vi "TwTpsGetModuleCodes.vi"(0 "error in (no error)":errorcluster) -> (1 "error out":errorcluster, 2 "moduleCodeBuffer":i32[](array[numeric]))   [LabVIEW 2009]
uses:
  Release_Build/TofDaqDll.dll
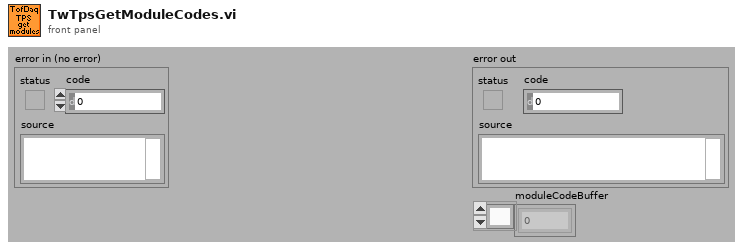
[diagram p1: front panel]
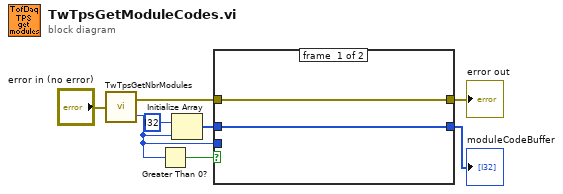
[diagram p0: block diagram]
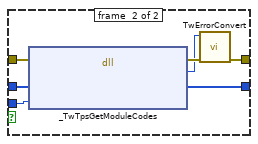
[diagram p2: hidden frame]
diagram:
  n1 = call "TwTpsGetNbrModules.vi"("error in (no error)"="error in (no error)") -> ("error out"=w6:errorcluster, "nbrModules"=w1:i32)
  n2 = Greater Than 0?(x=w1) -> (x > 0?=w2:bool)
  n3 = Initialize Array(i32 ? ("element"), w1) -> (w4:i32[])
  n4 = case shown="True" w2 {
    tunnel: [w9 w16] -> w8
    tunnel: w6 -> [w9 w14]
    tunnel: w4 -> [w10 w13]
    tunnel: w1 -> [_ w12]
    tunnel: [w10 w11] -> w3
    frame #0 {
    }
    frame #1 {
      n5 = dll-call lib="C:/src/TofDaq/Release_Build/TofDaqDll.dll" fn="_TwTpsGetModuleCodes"(error in=w14, "moduleCodeBuffer"=w13, "bufferLength"=w12) -> (error out=w17:errorcluster, "TwRetVal"=w15:i32, "moduleCodeBuffer"=w11:i32[])  [unwired: 3 in, 1 out]
      n6 = call "TwErrorConvert.vi"("error in (no error)"=w17, "error code"=w15) -> ("error out"=w16:errorcluster)  [unwired: 9 out]
    }
  }
  "error out" <- w8
  "moduleCodeBuffer" <- w3
